vi "Wrap Next Generation.vi"(8 "error in":errorcluster, 9 "Update Interval":u32, 10 "generation in":u32 caption="Generation", 11 "cells in":bool[][](array[boolean])) -> (0 "error out":errorcluster, 1 "game of life":T1, 2 "generation out":u32, 3 "cells out":bool[][](array[boolean]), 4 "Stop?":bool)   [LabVIEW 2021, in "Game of Life.lvlib"]
doc: "This VI generates the next generation of living cells by applying the game logic and convets them to XY coordinates of the game of life board."
uses:
  Game of Life.lvlib
  Game of Life.ctl
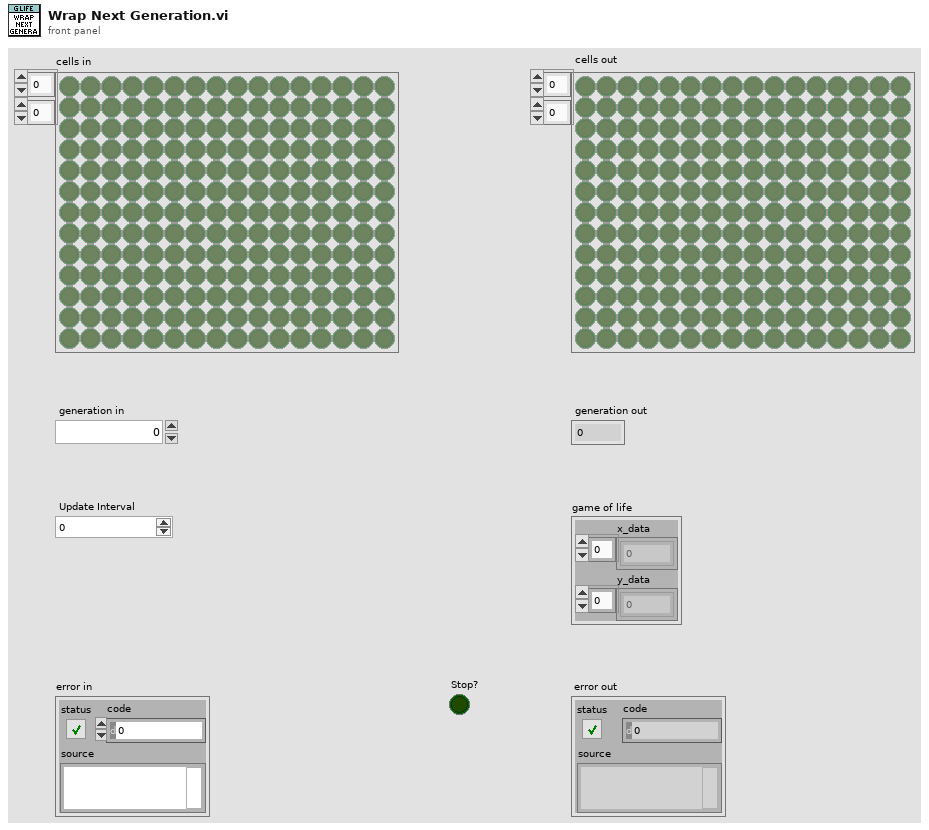
[diagram p1: front panel]
types:
  T1 = typedef "Game of Life.lvlib/Game of Life.ctl" = cluster{"x_data":dbl[], "y_data":dbl[]}
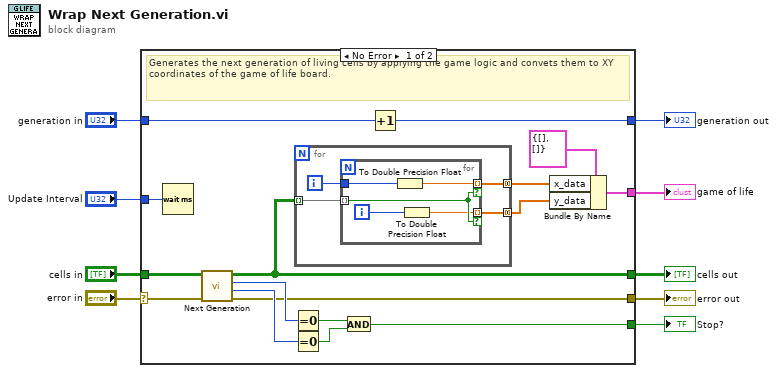
[diagram p0: block diagram]
diagram:
  n1 = case shown="No Error" "error in" {
    selector: "error in" -> [w25 w36]
    tunnel: "cells in" -> [w24 w35]
    tunnel: [w17 _] -> w5
    tunnel: "generation in" -> [w15 w37]
    tunnel: [w16 w36] -> w3
    tunnel: [w14 w37] -> w6
    tunnel: [w13 _] -> w1
    tunnel: [w12 w35] -> w4
    tunnel: "Update Interval" -> [w11 _]
    frame No Error {
      # "Generates the next generation of living cells by applying the game logic and convets them to XY coordinates of the game of life board."
      n2 = Wait (ms)(milliseconds to wait=w11) -> ()  [unwired: 1 out]
      n3 = call "Next Generation.vi"("error in"=w25, "cells in"=w24) -> ("error out"=w16:errorcluster, "deaths"=w20:i32, "births"=w21:i32, "cells out"=w12:bool[][])  [unwired: 6 in]
      n4 = Equal To 0?(x=w21) -> (x = 0?=w22:bool)
      n5 = Equal To 0?(x=w20) -> (x = 0?=w23:bool)
      n6 = for {
        tunnel: w12 -> [w29] mode=indexing
        tunnel: [w27] -> w19 mode=concatenating
        tunnel: [w26] -> w18 mode=concatenating
        i -> [w28]
        n7 = for {
          tunnel: w29 -> [w34] mode=indexing
          tunnel: [w32] -> w27 mode=indexing if=w34
          tunnel: w28 -> [w33]
          tunnel: [w30] -> w26 mode=indexing if=w34
          i -> [w31]
          n8 = To Double Precision Float(number=w33) -> (double precision float=w32:dbl)
          n9 = To Double Precision Float(number=w31) -> (double precision float=w30:dbl)
        }
      }
      n10 = And(x=w22, y=w23) -> (x .and. y?=w17:bool)
      n11 = Increment(x=w15) -> (x+1=w14:u32)
      n12 = Bundle By Name(cluster=T1 {"x_data"=[], "y_data"=[]} ("game of life"), "x_data"=w19, "y_data"=w18) -> (w13:T1)
    }
    frame Error {
    }
  }
  "generation out" <- w6
  "Stop?" <- w5
  "cells out" <- w4
  "error out" <- w3
  "game of life" <- w1
